vi "通过模板匹配找螺帽中心.vi"(9 "量测规格":T3 {"上限" format="%#.4g"; "下限" format="%#.4g"}, 11 "Img输入":T1) -> (0 "Fitted Circle":T2, 1 "Radius (Pixels)":dbl, 2 "在规格内":bool, 3 "Img输入 out":T1)   [LabVIEW 2014]
uses:
  <vilib>/vision/Image Controls.llb/IMAQ Image.ctl
  Controls/TestThreshold.ctl
  Global.vi
panel:
  # "~"
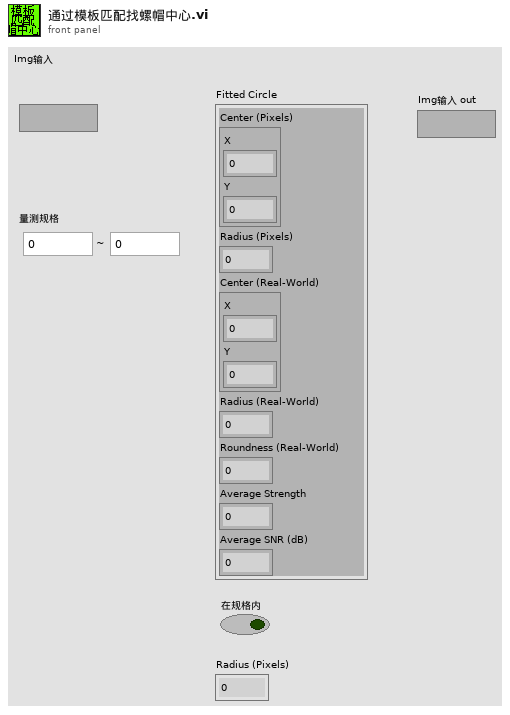
[diagram p1: front panel]
types:
  T1 = typedef "IMAQ Image.ctl" = refnum<image>
  T2 = cluster{"Center (Pixels)":cluster{"X":sgl, "Y":sgl}, "Radius (Pixels)":dbl, "Center (Real-World)":cluster{"X":sgl, "Y":sgl}, "Radius (Real-World)":dbl, "Roundness (Real-World)":dbl, "Average Strength":dbl, "Average SNR (dB)":dbl}
  T3 = typedef "TestThreshold.ctl" = cluster{"下限":dbl, "上限":dbl}
  T4 = typedef "OtherSpec.ctl" = cluster{"其它勾选类规格":T5, "其它数据类规格":T6, "相机名称":T7, "参数":cluster{"Mark1曝光时间":i32, "Mark2曝光时间":i32, "二维码曝光时间":i32}}
  T5 = typedef "其它勾选类规格.ctl" = cluster{"保存图片":bool, "上传设备状态数据":bool, "保存数据":bool, "开机默认开启监控摄像头":bool, "启用mark拍照 ":bool}
  T6 = typedef "其他数据类规格.ctl" = cluster{"相机1像素-毫米换算系数":dbl, "相机2像素-毫米换算系数":dbl, "D盘剩余空间预警(G)":dbl, "视频最长录制时间(秒)":dbl}
  T7 = typedef "相机名称品牌使用状态.ctl" = cluster{"相机1名称":T8, "相机2名称":T8, "Cam1启用":bool, "Cam2启用":bool, "Basler1":bool, "Basler2":bool}
  T8 = typedef "IMAQdx.ctl" = refnum<k21>
  T9 = cluster{"Position":cluster{"x":sgl, "y":sgl}, "Angle":sgl, "Scale":sgl, "Score":sgl, "Bounding Box":cluster{"x":sgl, "y":sgl}[]}[]
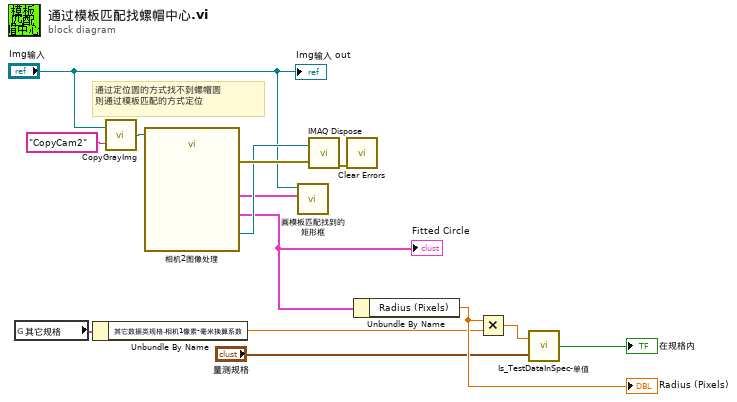
[diagram p0: block diagram]
diagram:
  # "通过定位圆的方式找不到螺帽圆\n则通过模板匹配的方式定位"
  n1 = global read "Global.vi" "其它规格"() -> (w2:T4)
  n2 = Unbundle By Name(w2) -> ("其它数据类规格.相机1像素-毫米换算系数"=w1:dbl)
  n3 = call "CopyGrayImg.vi"("Image Name"="CopyCam2", "Image In"="Img输入") -> ("Image Out"=w6:T1)
  n4 = call "相机2图像处理"("Image In"=w6) -> ("Image Out"=w10:T1, "Matches (Pattern Matching 1)"=w4:T9, "Fitted Circle (Find Circular Edge 1)"=w3:T2, "error out"=w11:errorcluster)  [unwired: 23 in]
  "Fitted Circle" <- w3
  n5 = call "画模板匹配找到的矩形框.vi"("Matches (Pattern Matching 1)"=w4, "Image"="Img输入") -> ()  [unwired: 10 in]
  n6 = call "IMAQ Dispose"("Image"=w10, "error in (no error)"=w11) -> ("error out"=w12:errorcluster)  [unwired: 4 in]
  n7 = call <vilib>:"Clear Errors.vi"("error in (no error)"=w12) -> ()  [unwired: 5 in, 2 out]
  n8 = Unbundle By Name(w3) -> ("Radius (Pixels)"=w13:dbl)
  "Radius (Pixels)" <- w13
  n9 = Multiply(x=w13, y=w1) -> (x*y=w14:dbl)
  n10 = call "Is_TestDataInSpec-单值.vi"("量测规格"="量测规格", "相机量测结果"=w14) -> ("在规格内"=→"在规格内":bool)
  "Img输入 out" <- "Img输入"
